vi "Get Name Or Data Format As String.vi"(8 "error in (no error)":errorcluster, 10 "Data":variant) -> (0 "error out":errorcluster, 2 "Data Value OR Name":string)   [LabVIEW 2013, in "VITesterUtilities.lvlib"]
uses:
  Libraries/VITesterUtilities.lvlib
  JKI Reuse/Filter Error Codes (Scalar)__jki_lib_error_handling -- VI Tester.vi
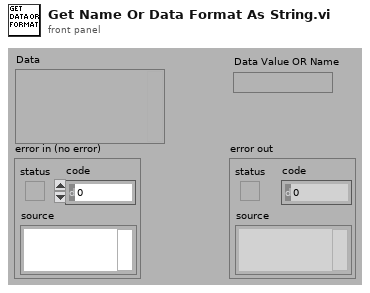
[diagram p1: front panel]
types:
  T1 = typedef "Type Descriptor Enumeration__ogtk.ctl" = enum8{"<Null>", "I8", "I16", "I32", "I64", "U8", "U16", "U32", "U64", "SGL", "DBL", "EXT", "CSG", "CDB", "CXT", "0x0F", "0x10", "0x11", "0x12", "0x13", "0x14", "Enum U8", "Enum U16", "Enum U32", "Enum U64", "SGL PQ", "DBL PQ", "EXT PQ", "CSG PQ", "CDB PQ", "CXT PQ", "0x1F", "0x20", "Boolean", "0x22", "0x23", "0x24", "0x25", "0x26", "0x27", "0x28", "0x29", "0x2A", "0x2B", "0x2C", "0x2D", "0x2E", "0x2F", "String", "0x31", "Path", "Pict", "0x34", "0x35", "0x36", "DAQ", "0x38", "0x39", "0x3A", "0x3B", "0x3C", "0x3D", "0x3E", "0x3F", "Array", "0x41", "0x42", "0x43", "0x44", "0x45", "0x46", "0x47", "0x48", "0x49", "0x4A", "0x4B", "0x4C", "0x4D", "0x4E", "0x4F", "Cluster", "0x51", "0x52", "Variant", "Waveform", "0x55", "0x56", "0x57", "0x58", "0x59", "0x5A", "0x5B", "0x5C", "0x5D", "0x5E", "0x5F", "0x60", "0x61", "0x62", "0x63", "0x64", "0x65", "0x66", "0x67", "0x68", "0x69", "0x6A", "0x6B", "0x6C", "0x6D", "0x6E", "0x6F", "Refnum"}
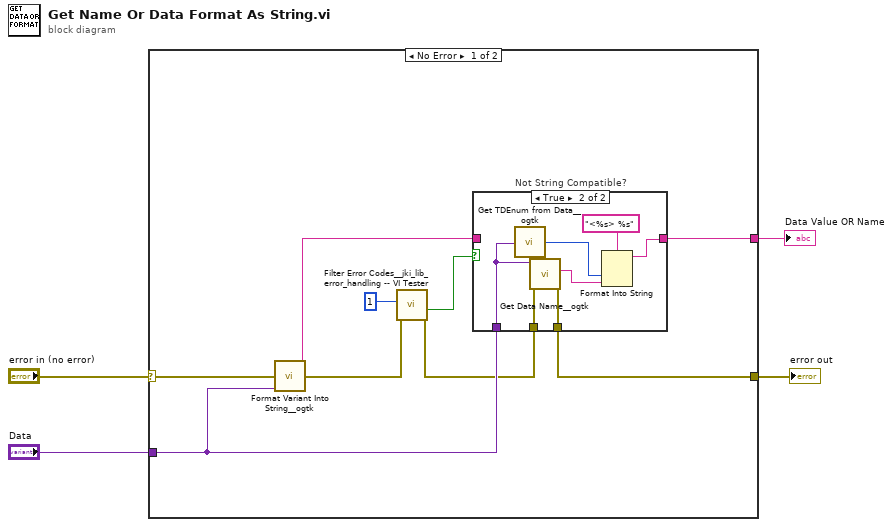
[diagram p0: block diagram]
diagram:
  n1 = case shown="No Error" "error in (no error)" {
    selector: "error in (no error)" -> [w13 w23]
    tunnel: [w5 w23] -> w4
    tunnel: "Data" -> [w7 _]
    tunnel: [w9 _] -> w1
    frame No Error {
      n2 = call <userlib>:"Format Variant Into String__ogtk.vi"("error in (no error)"=w13, "Variant"=w7) -> ("Output String"=w8:string, "error out"=w12:errorcluster)  [unwired: 12 in]
      n3 = call-poly "Filter Error Codes__jki_lib_error_handling -- VI Tester.vi"("error in"=w12, "error code to filter"=1) -> ("error out"=w6:errorcluster, "error filtered?"=w10:bool)  [unwired: 7 in, 1 out]
      n4 = case "Not String Compatible?" shown="True" w10 {
        tunnel: [w15 w16] -> w9
        tunnel: w8 -> [w15 _]
        tunnel: w7 -> [_ w22]
        tunnel: w6 -> [w14 w21]
        tunnel: [w14 w20] -> w5
        frame False {
        }
        frame True {
          n5 = call <userlib>:"Get TDEnum from Data__ogtk.vi"("Data"=w22) -> ("Type Descriptor Enumeration"=w19:T1)  [unwired: 4 in]
          n6 = call <userlib>:"Get Data Name__ogtk.vi"("error in (no error)"=w21, "Data"=w22) -> ("error out"=w20:errorcluster, "Data Name"=w18:string)  [unwired: 7 in, 1 out]
          n7 = Format Into String(format string="<%s> %s", w19, w18) -> (resulting string=w16:string)  [unwired: 2 in, 1 out]
        }
      }
    }
    frame Error {
    }
  }
  "error out" <- w4
  "Data Value OR Name" <- w1
